vi "start.vi"(8 "error in (no error)":errorcluster, 11 "librarian_sm in":refnum<class "librarian.lvclass">) -> (0 "error out":errorcluster, 3 "librarian_sm out":refnum<class "librarian.lvclass">)   [LabVIEW 2020, in "librarian.lvclass"]
uses:
  librarian.lvclass
  main.vi
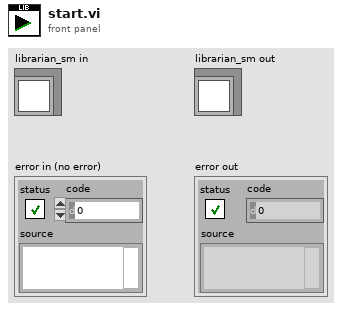
[diagram p1: front panel]
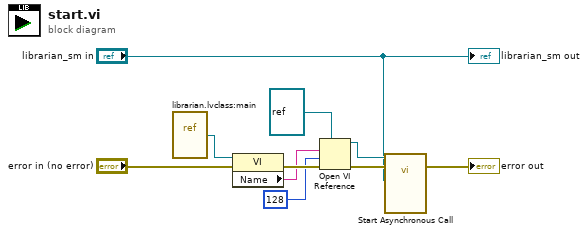
[diagram p0: block diagram]
diagram:
  n1 = vi-ref "librarian.lvclass:main.vi"() -> (w10:refnum<vi>)
  n2 = property class="VI"(reference=w10, error in="error in (no error)") -> (error out=w8:errorcluster, "Name"=w7:string)  [unwired: 1 out]
  n3 = Open VI Reference(type specifier VI Refnum (for type only)=refnum<vi> refnum ("reference"), vi path=w7, options=128, error in (no error)=w8) -> (vi reference=w3:refnum<vi>, error out=w4:errorcluster)  [unwired: 2 in]
  n4 = call-by-ref "Start Asynchronous Call"(reference=w3, error in=w4, "librarian_sm.lvclass"="librarian_sm in") -> (error out=→"error out":errorcluster)  [unwired: 11 in, 1 out]
  "librarian_sm out" <- "librarian_sm in"
